vi "Calculate defocus.vi"(8 "error in (no error)":errorcluster, 11 "Retiga in":refnum<class "Retiga.lvclass">) -> (0 "error out":errorcluster, 1 "fine?":bool, 2 "translation out":dbl[unit], 3 "Retiga out":refnum<class "Retiga.lvclass">)   [LabVIEW 2012, in "Retiga.lvclass"]
uses:
  Retiga.lvclass
  dependencies/ImageReg/Registration method.ctl
  Retiga.lvclass/Retiga.ctl
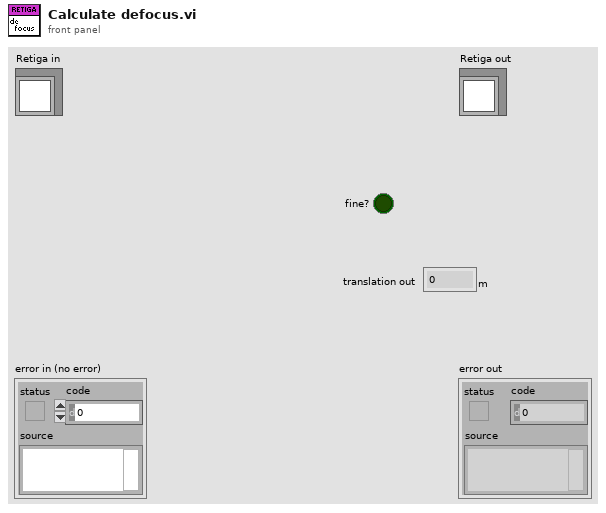
[diagram p1: front panel]
types:
  T1 = typedef "Registration method.ctl" = enum16{"Binarization", "Difference of Gaussians", "Edges Detection", "Gaussians and Binarization", "Edges and Gaussians", "Edges and Binarization", "All"}
  T2 = typedef "IMAQ Image.ctl" = refnum<image>
  T3 = typedef "BinarizationParameters.ctl" = cluster{"threshold percentage":dbl, "equalize?":bool, "Method (clustering)":i32}
  T4 = typedef "Gaussian blur parameters.ctl" = cluster{"large sigma":sgl, "small sigma":sgl, "equalize?":bool}
  T5 = typedef "Edge and object parameters.ctl" = cluster{"Canny Edge Parameters":cluster{"Sigma":sgl, "HThresh":sgl, "LThres":sgl, "WindowSize":i32}, "Smoothing parameters":cluster{"X Size":i32, "Y Size":i32, "% Tolerance":i32}, "Dilation iteration":i32, "Object recognition parameters":cluster{"Objects":u16, "Threshold":i32, "Reject Border":bool, "Fill Holes":bool, "Min Object Size":bool, "Min Size":i32, "Max Object Size":bool, "Max Size":i32, "Show Search Area":bool, "Show Center":bool, "Show Bounding Box":bool}}
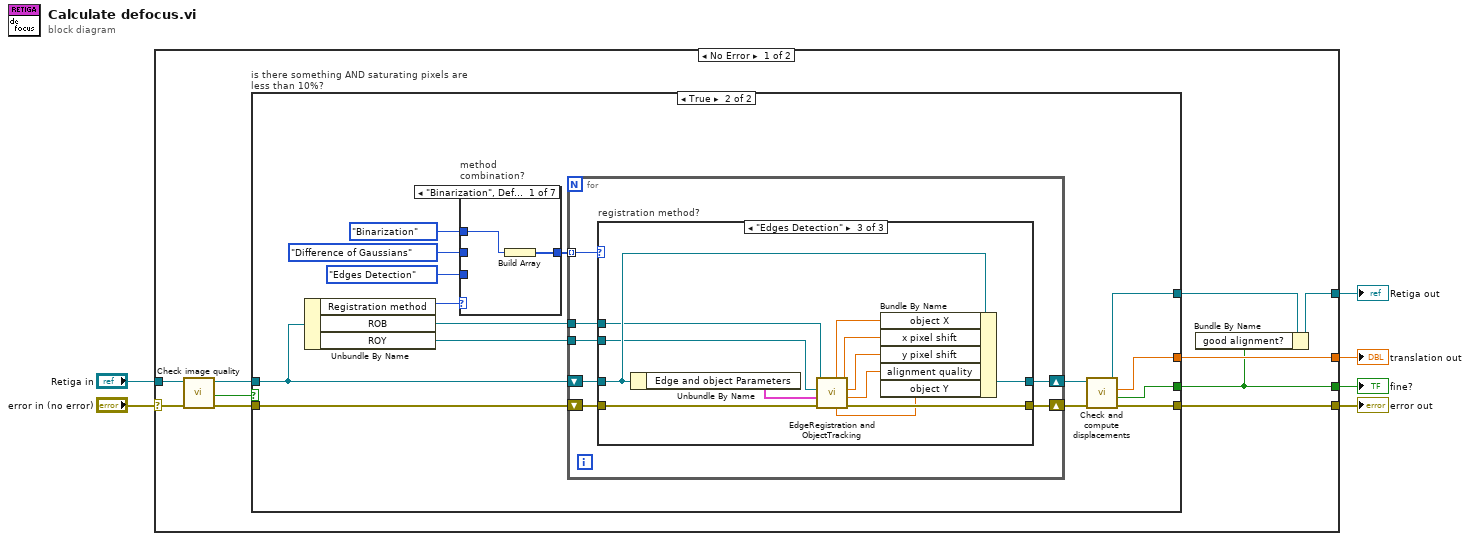
[diagram p0: block diagram]
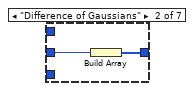
[diagram p3: hidden frame]
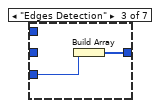
[diagram p4: hidden frame]
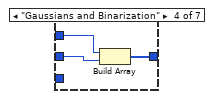
[diagram p5: hidden frame]
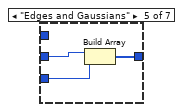
[diagram p6: hidden frame]
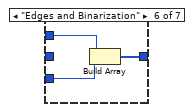
[diagram p7: hidden frame]
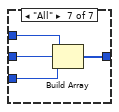
[diagram p8: hidden frame]
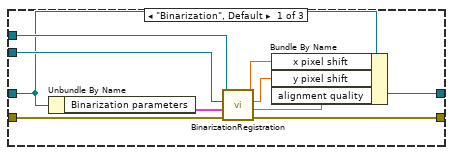
[diagram p9: hidden frame]
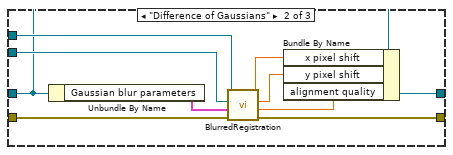
[diagram p10: hidden frame]
diagram:
  n1 = case shown="No Error" "error in (no error)" {
    selector: "error in (no error)" -> [w13 w93]
    tunnel: [w14 w93] -> w5
    tunnel: [w15 w92] -> w3
    tunnel: "Retiga in" -> [w10 w92]
    tunnel: [w7 _] -> w2
    tunnel: [w8 _] -> w1
    frame No Error {
      n2 = call-dynamic "Check image quality.vi"("error in (no error)"=w13, "Retiga in"=w10) -> ("error out"=w12:errorcluster, "QC passed?"=w11:bool, "Retiga out"=w9:refnum<class "Retiga.lvclass">)  [unwired: 7 in]
      n3 = case "is there something AND saturating pixels are less than 10%?" shown="True" w11 {
        tunnel: [w18 w26] -> w16
        tunnel: [w17 w27] -> w14
        tunnel: w9 -> [w18 w33]
        tunnel: w12 -> [w17 w32]
        tunnel: [_ w25] -> w7
        tunnel: [_ w24] -> w8
        frame False {
        }
        frame True {
          n4 = Unbundle By Name(w33) -> ("Registration method"=w23:T1, "ROB"=w31:T2, "ROY"=w30:T2)
          n5 = case "method\ncombination?" shown="\"Binarization\", Default" w23 {
            tunnel: [w35 w37 w39 w42 w45 w48 w52] -> w22
            tunnel: Registration_method."Difference of Gaussians" ("Registration method") -> [_ w36 _ w40 w44 _ w49]
            tunnel: Registration_method."Binarization" ("Registration method") -> [w34 _ _ w41 _ w46 w51]
            tunnel: Registration_method."Edges Detection" ("Registration method") -> [_ _ w38 _ w43 w47 w50]
            frame "Binarization", Default {
              n6 = Build Array(w34) -> (w35:T1[])
            }
            frame "Difference of Gaussians" {
              n7 = Build Array(w36) -> (w37:T1[])
            }
            frame "Edges Detection" {
              n8 = Build Array(w38) -> (w39:T1[])
            }
            frame "Gaussians and Binarization" {
              n9 = Build Array(w41, w40) -> (w42:T1[])
            }
            frame "Edges and Gaussians" {
              n10 = Build Array(w44, w43) -> (w45:T1[])
            }
            frame "Edges and Binarization" {
              n11 = Build Array(w46, w47) -> (w48:T1[])
            }
            frame "All" {
              n12 = Build Array(w51, w49, w50) -> (w52:T1[])
            }
          }
          n13 = for {
            tunnel: w31 -> [w57]
            tunnel: w30 -> [w56]
            shift-right: [w54] -> w28
            shift-left: w33 -> [w59]
            shift-right: [w55] -> w29
            shift-left: w32 -> [w58]
            tunnel: w22 -> [w53] mode=indexing
            n14 = case "registration method?" shown="\"Edges Detection\"" w53 {
              tunnel: w59 -> [w65 w75 w91]
              tunnel: w58 -> [w69 w79 w89]
              tunnel: w57 -> [w68 w78 w85]
              tunnel: w56 -> [w67 w77 w86]
              tunnel: [w64 w71 w88] -> w55
              tunnel: [w63 w70 w90] -> w54
              frame "Binarization", Default {
                n15 = Unbundle By Name(w65) -> ("Binarization parameters"=w66:T3)
                n16 = call "BinarizationRegistration.vi"("error in"=w69, "Binarization parameters"=w66, "Roy"=w67, "Rob"=w68) -> ("error out"=w64:errorcluster, "quality"=w62:dbl, "y translation"=w61:dbl, "x translation"=w60:dbl)  [unwired: 4 in]
                n17 = Bundle By Name(cluster=w65, "x pixel shift"=w60, "y pixel shift"=w61, "alignment quality"=w62) -> (w63:refnum<class "Retiga.lvclass">)
              }
              frame "Difference of Gaussians" {
                n18 = Unbundle By Name(w75) -> ("Gaussian blur parameters"=w76:T4)
                n19 = call "BlurredRegistration.vi"("error in"=w79, "Gaussian blur parameters"=w76, "roy"=w77, "rob"=w78) -> ("error out"=w71:errorcluster, "alignment quality"=w72:dbl, "y displacement"=w73:dbl, "x displacement"=w74:dbl)  [unwired: 4 in]
                n20 = Bundle By Name(cluster=w75, "x pixel shift"=w74, "y pixel shift"=w73, "alignment quality"=w72) -> (w70:refnum<class "Retiga.lvclass">)
              }
              frame "Edges Detection" {
                n21 = Unbundle By Name(w91) -> ("Edge and object Parameters"=w87:T5)
                n22 = call "EdgeRegistration and ObjectTracking.vi"("error in (no error)"=w89, "Edge and object Parameters"=w87, "Roy"=w86, "Rob"=w85) -> ("error out"=w88:errorcluster, "Max value"=w84:dbl, "y translation"=w83:dbl, "x translation"=w82:dbl, "object center y"=w80:sgl, "object center X"=w81:sgl)  [unwired: 2 in]
                n23 = Bundle By Name(cluster=w91, "object X"=w81, "x pixel shift"=w82, "y pixel shift"=w83, "alignment quality"=w84, "object Y"=w80) -> (w90:refnum<class "Retiga.lvclass">)
              }
            }
          }
          n24 = call-dynamic "Check and compute displacements.vi"("error in (no error)"=w29, "Retiga in"=w28) -> ("error out"=w27:errorcluster, "fine?"=w25:bool, "translation out"=w24:dbl[unit], "Retiga out"=w26:refnum<class "Retiga.lvclass">)  [unwired: 6 in]
        }
      }
      n25 = Bundle By Name(cluster=w16, "good alignment?"=w7) -> (w15:refnum<class "Retiga.lvclass">)
    }
    frame Error {
    }
  }
  "error out" <- w5
  "Retiga out" <- w3
  "fine?" <- w2
  "translation out" <- w1
